vi "start.vi"(10 "Device Reference in":T1 format="%.0x", 11 "state in":T2) -> (0 "code":i32, 3 "state out":T2)   [LabVIEW 2015, in "Scriptable Model Interface Engine.lvlib"]
uses:
  Scriptable Model Interface Engine.lvlib
  runtime state.ctl
  Shared/model parameters.ctl
  <vilib>/NI Veristand/Custom Device API/Custom Device Item Ref.ctl
  <vilib>/NI Veristand/Custom Device API/Custom Device API.lvlib
  Shared/Scriptable Model Interface Shared.lvlib
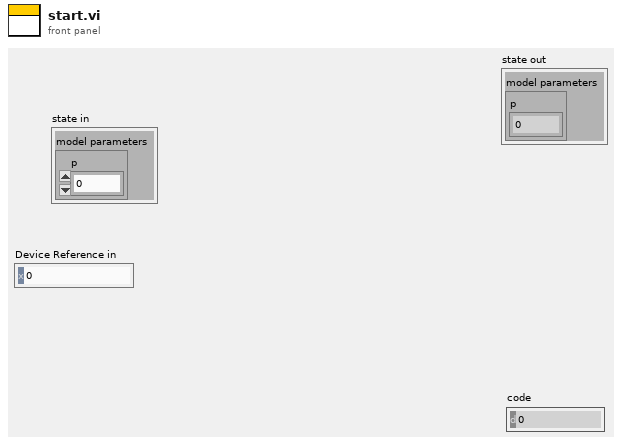
[diagram p1: front panel]
types:
  T1 = typedef "Custom Device API.lvlib/Custom Device Item Ref.ctl" = u64
  T2 = typedef "Scriptable Model Interface Engine.lvlib/runtime state.ctl" = cluster{"model parameters":T3}
  T3 = typedef "Scriptable Model Interface Shared.lvlib/model parameters.ctl" = cluster{"p":dbl}
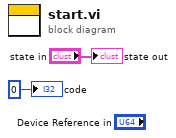
[diagram p0: block diagram]
diagram:
  "state out" <- "state in"
  "code" <- 0 ("code")
